vi "Global indicator.vi"() -> ()   [LabVIEW 2018]
uses:
  Global 1.vi
panel:
  out "Numeric":dbl
  out "String":string
  out "Boolean":bool
  in  "stop":bool
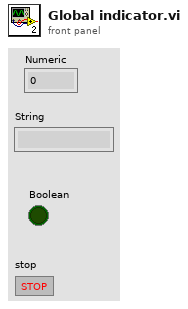
[diagram p1: front panel]
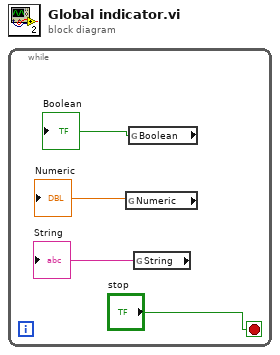
[diagram p0: block diagram]
diagram:
  n1 = while {
    stop <- "stop" stop-if-true
    n2 = global read "Global 1.vi" "Numeric"() -> (→"Numeric":dbl)
    n3 = global read "Global 1.vi" "Boolean"() -> (→"Boolean":bool)
    n4 = global read "Global 1.vi" "String"() -> (→"String":string)
  }
